vi "TDMSAdv init.vi"(8 "error in (no error)":errorcluster, 11 "TDMSAdv in":refnum<class "TDMSAdv.lvclass">) -> (0 "error out":errorcluster, 3 "TDMSAdv out":refnum<class "TDMSAdv.lvclass">)   [LabVIEW 2018, in "TDMSAdv.lvclass"]
uses:
  TDMSAdv.lvclass
  TDMSAdv.lvclass/TDMSAdv.ctl
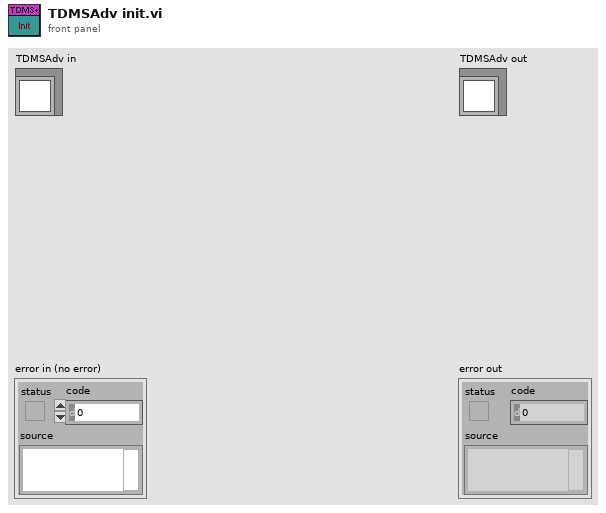
[diagram p1: front panel]
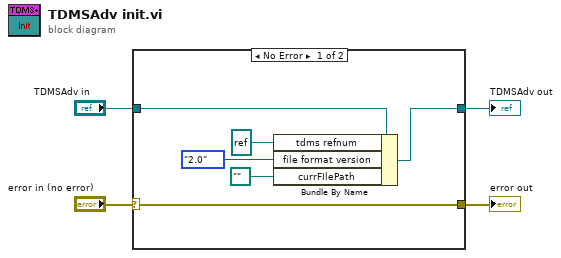
[diagram p0: block diagram]
diagram:
  n1 = case shown="No Error" "error in (no error)" {
    selector: "error in (no error)" -> [w10 w12]
    tunnel: [w10 w12] -> w3
    tunnel: [w6 w11] -> w1
    tunnel: "TDMSAdv in" -> [w9 w11]
    frame No Error {
      n2 = Bundle By Name(cluster=w9, "tdms refnum"=refnum<k34> refnum, "file format version"=enum16{"1.0", "2.0", "Adv"}."2.0", "currFIlePath"=path "") -> (w6:refnum<class "TDMSAdv.lvclass">)
    }
    frame Error {
    }
  }
  "error out" <- w3
  "TDMSAdv out" <- w1
